vi "ta_calc_diff.vi"(0 "data in":dbl[][](array[numeric]), 9 "ref in":dbl[][](array[numeric]), 11 "Algorithm":T1=3 items=["<(S*-S)/S>/ln(10)", "<S*/S>-1", "<S*/PD*>/<S/PD>", "<S*/Sref*>/<S/Sref>", "<S*/Sref*/PD*>/<S/Sref>", "<S*/Sref*>/<S/Sref>_alt"], 12 "PD values in":dbl[][](array[numeric])) -> (1 "pumped std":dbl[](array[numeric]), 3 "unpumped std":dbl[](array[numeric]), 4 "pumped":dbl[](array[numeric]), 6 "unpumped":dbl[](array[numeric]), 8 "diff std":dbl[](array[numeric]), 10 "diff":dbl[](array[numeric]), 14 "ref std":dbl[](array[numeric]), 15 "ref mean":dbl[](array[numeric]))   [LabVIEW 2019]
uses:
  data_algorithm.ctl
  <vilib>/Analysis/baseanly.llb/Mean (DBL).vi
  <vilib>/Analysis/NI_AALBase.lvlib
panel:
  out "size data":i32[](array[numeric])
  out "size ref":i32[](array[numeric])
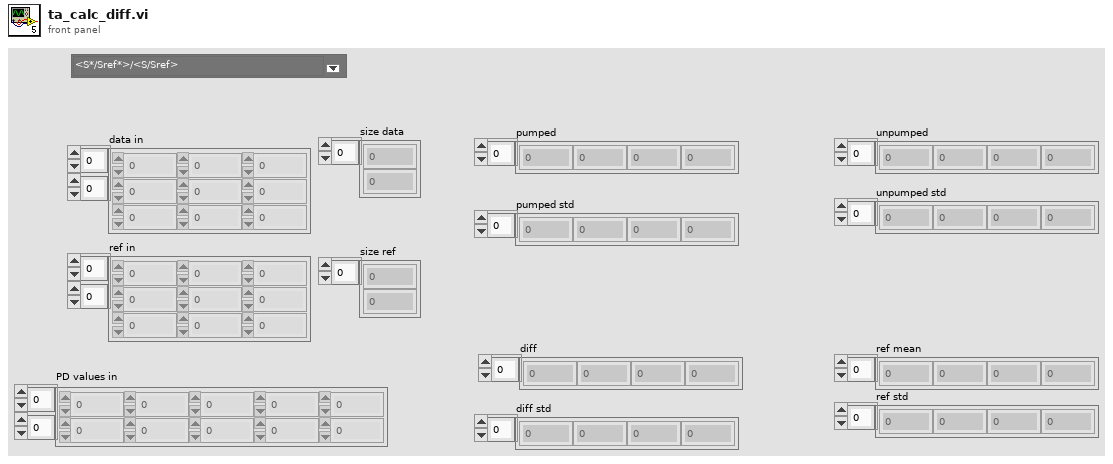
[diagram p1: front panel]
types:
  T1 = typedef "data_algorithm.ctl" = u16
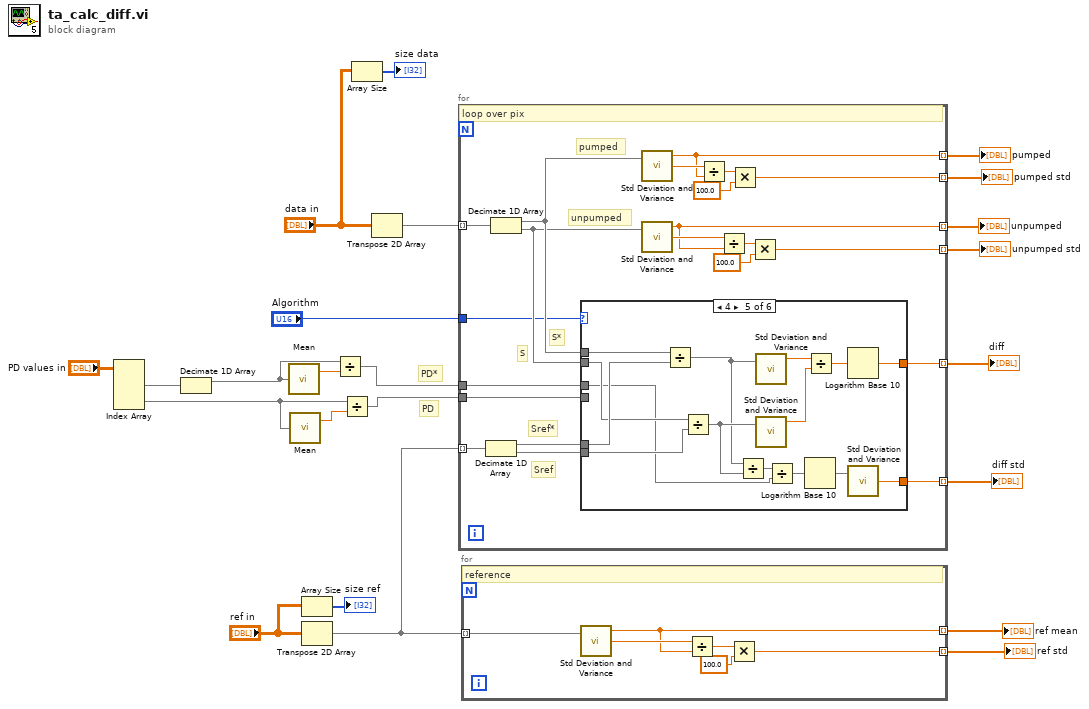
[diagram p0: block diagram]
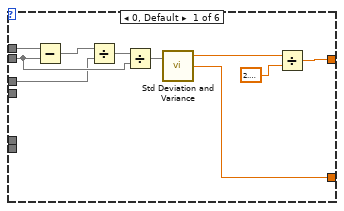
[diagram p2: hidden frame]
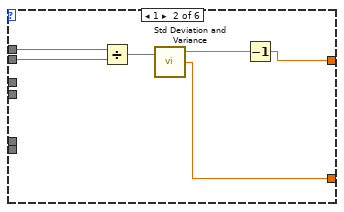
[diagram p3: hidden frame]
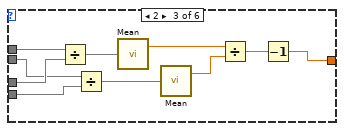
[diagram p4: hidden frame]
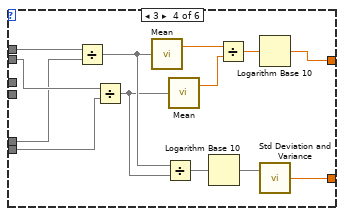
[diagram p5: hidden frame]
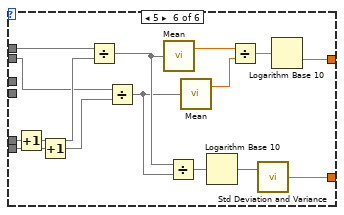
[diagram p6: hidden frame]
diagram:
  # "PD"
  # "PD*"
  n1 = Index Array(array="PD values in") -> (element #1=w3:dbl[], element #2=w6:dbl[])  [unwired: 4 in]
  n2 = Decimate 1D Array(w3) -> (w2:dbl[])  [unwired: 1 out]
  n3 = call-poly <vilib>:"Mean.vi"("X"=w2) -> ("mean"=w7:dbl)  [unwired: 1 out]
  n4 = call-poly <vilib>:"Mean.vi"("X"=w6) -> ("mean"=w5:dbl)  [unwired: 1 out]
  n5 = Array Size(array="ref in") -> (size(s)=→"size ref":i32[])
  n6 = Transpose 2D Array(2D array="ref in") -> (transposed array=w11:dbl[][])
  n7 = Divide(x=w2, y=w7) -> (x/y=w8:dbl[])
  n8 = Divide(x=w6, y=w5) -> (x/y=w4:dbl[])
  n9 = Array Size(array="data in") -> (size(s)=→"size data":i32[])
  n10 = Transpose 2D Array(2D array="data in") -> (transposed array=w17:dbl[][])
  n11 = for {
    tunnel: w17 -> [w42] mode=indexing
    tunnel: [w33] -> w23 mode=indexing
    tunnel: [w40] -> w22 mode=indexing
    tunnel: [w37] -> w15 mode=indexing
    tunnel: [w32] -> w14 mode=indexing
    tunnel: "Algorithm" -> [w31]
    tunnel: [w30] -> w12 mode=indexing
    tunnel: w8 -> [w25]
    tunnel: w4 -> [w29]
    tunnel: w11 -> [w28] mode=indexing
    tunnel: [w24] -> w1 mode=indexing
    # "Sref"
    # "Sref*"
    # "S"
    # "S*"
    # "unpumped"
    # "pumped"
    # "loop over pix"
    n12 = Decimate 1D Array(w28) -> (w27:dbl[], w26:dbl[])
    n13 = Decimate 1D Array(w42) -> (w44:dbl[], w43:dbl[])
    n14 = case shown="4" w31 {
      tunnel: w44 -> [w54 w60 w70 w83 w96 w107]
      tunnel: w43 -> [w53 w59 w68 w82 w94 w106]
      tunnel: [w49 w58 w61 w77 w97 w108] -> w30
      tunnel: w25 -> [w50 _ w69 _ w85 _]
      tunnel: w29 -> [_ _ w67 _ _ _]
      tunnel: w27 -> [_ _ _ w76 w95 w105]
      tunnel: w26 -> [_ _ _ w81 w93 w104]
      tunnel: [w47 w55 _ w71 w88 w99] -> w24
      frame 0, Default {
        n15 = Subtract(x=w54, y=w53) -> (x-y=w46:dbl[])
        n16 = Divide(x=w46, y=w50) -> (x/y=w51:dbl[])
        n17 = Divide(x=w51, y=w53) -> (x/y=w45:dbl[])
        n18 = call <vilib>:"Std Deviation and Variance.vi"("X"=w45) -> ("mean"=w48:dbl, "standard deviation"=w47:dbl)  [unwired: 1 in, 1 out]
        n19 = Divide(x=w48, y=2.302585092994046) -> (x/y=w49:dbl)
      }
      frame 1 {
        n20 = Divide(x=w60, y=w59) -> (x/y=w57:dbl[])
        n21 = call <vilib>:"Std Deviation and Variance.vi"("X"=w57) -> ("mean"=w56:dbl, "standard deviation"=w55:dbl)  [unwired: 1 in, 1 out]
        n22 = Decrement(x=w56) -> (x-1=w58:dbl)
      }
      frame 2 {
        n23 = Divide(x=w70, y=w69) -> (x/y=w66:dbl[])
        n24 = Divide(x=w68, y=w67) -> (x/y=w65:dbl[])
        n25 = call-poly <vilib>:"Mean.vi"("X"=w66) -> ("mean"=w64:dbl)  [unwired: 1 out]
        n26 = call-poly <vilib>:"Mean.vi"("X"=w65) -> ("mean"=w63:dbl)  [unwired: 1 out]
        n27 = Divide(x=w64, y=w63) -> (x/y=w62:dbl)
        n28 = Decrement(x=w62) -> (x-1=w61:dbl)
      }
      frame 3 {
        n29 = Divide(x=w83, y=w76) -> (x/y=w75:dbl[])
        n30 = Divide(x=w82, y=w81) -> (x/y=w74:dbl[])
        n31 = call-poly <vilib>:"Mean.vi"("X"=w75) -> ("mean"=w80:dbl)  [unwired: 1 out]
        n32 = Divide(x=w75, y=w74) -> (x/y=w73:dbl[])
        n33 = call-poly <vilib>:"Mean.vi"("X"=w74) -> ("mean"=w79:dbl)  [unwired: 1 out]
        n34 = Logarithm Base 10(1:w73) -> (0:w72:dbl[])
        n35 = Divide(x=w80, y=w79) -> (x/y=w78:dbl)
        n36 = Logarithm Base 10(1:w78) -> (0:w77:dbl)
        n37 = call <vilib>:"Std Deviation and Variance.vi"("X"=w72) -> ("standard deviation"=w71:dbl)  [unwired: 1 in, 2 out]
      }
      frame 4 {
        n38 = Divide(x=w96, y=w95) -> (x/y=w87:dbl[])
        n39 = Divide(x=w94, y=w93) -> (x/y=w90:dbl[])
        n40 = Divide(x=w87, y=w90) -> (x/y=w86:dbl[])
        n41 = call <vilib>:"Std Deviation and Variance.vi"("X"=w87) -> ("mean"=w92:dbl)  [unwired: 1 in, 2 out]
        n42 = call <vilib>:"Std Deviation and Variance.vi"("X"=w90) -> ("mean"=w91:dbl)  [unwired: 1 in, 2 out]
        n43 = Divide(x=w86, y=w85) -> (x/y=w84:dbl[])
        n44 = Logarithm Base 10(1:w84) -> (0:w89:dbl[])
        n45 = Divide(x=w92, y=w91) -> (x/y=w98:dbl)
        n46 = Logarithm Base 10(1:w98) -> (0:w97:dbl)
        n47 = call <vilib>:"Std Deviation and Variance.vi"("X"=w89) -> ("standard deviation"=w88:dbl)  [unwired: 1 in, 2 out]
      }
      frame 5 {
        n48 = Increment(x=w105) -> (x+1=w112:dbl[])
        n49 = Increment(x=w104) -> (x+1=w113:dbl[])
        n50 = Divide(x=w107, y=w112) -> (x/y=w103:dbl[])
        n51 = Divide(x=w106, y=w113) -> (x/y=w102:dbl[])
        n52 = call-poly <vilib>:"Mean.vi"("X"=w103) -> ("mean"=w109:dbl)  [unwired: 1 out]
        n53 = Divide(x=w103, y=w102) -> (x/y=w101:dbl[])
        n54 = call-poly <vilib>:"Mean.vi"("X"=w102) -> ("mean"=w110:dbl)  [unwired: 1 out]
        n55 = Logarithm Base 10(1:w101) -> (0:w100:dbl[])
        n56 = Divide(x=w109, y=w110) -> (x/y=w111:dbl)
        n57 = call <vilib>:"Std Deviation and Variance.vi"("X"=w100) -> ("standard deviation"=w99:dbl)  [unwired: 1 in, 2 out]
        n58 = Logarithm Base 10(1:w111) -> (0:w108:dbl)
      }
    }
    n59 = call <vilib>:"Std Deviation and Variance.vi"("X"=w44) -> ("mean"=w40:dbl, "standard deviation"=w41:dbl)  [unwired: 1 in, 1 out]
    n60 = call <vilib>:"Std Deviation and Variance.vi"("X"=w43) -> ("mean"=w33:dbl, "standard deviation"=w34:dbl)  [unwired: 1 in, 1 out]
    n61 = Divide(x=w41, y=w40) -> (x/y=w39:dbl)
    n62 = Divide(x=w34, y=w33) -> (x/y=w36:dbl)
    n63 = Multiply(x=w39, y=100.0) -> (x*y=w37:dbl)
    n64 = Multiply(x=w36, y=100.0) -> (x*y=w32:dbl)
  }
  "diff" <- w12
  "unpumped" <- w23
  "pumped" <- w22
  "pumped std" <- w15
  "unpumped std" <- w14
  "diff std" <- w1
  n65 = for {
    tunnel: w11 -> [w119] mode=indexing
    tunnel: [w117] -> w21 mode=indexing
    tunnel: [w114] -> w16 mode=indexing
    # "reference"
    n66 = call <vilib>:"Std Deviation and Variance.vi"("X"=w119) -> ("mean"=w117:dbl, "standard deviation"=w118:dbl)  [unwired: 1 in, 1 out]
    n67 = Divide(x=w118, y=w117) -> (x/y=w116:dbl)
    n68 = Multiply(x=w116, y=100.0) -> (x*y=w114:dbl)
  }
  "ref mean" <- w21
  "ref std" <- w16
